vi "Is Dispense Boolean.vi"(8 "error in (no error)":errorcluster, 11 "Dispense in":refnum<class "Dispense.lvclass">) -> (0 "error out":errorcluster, 2 "Is Dispense?":bool, 3 "Dispense out":refnum<class "Dispense.lvclass">)   [LabVIEW 2016, in "Dispense.lvclass"]
uses:
  Dispense.lvclass
  Routine.lvclass
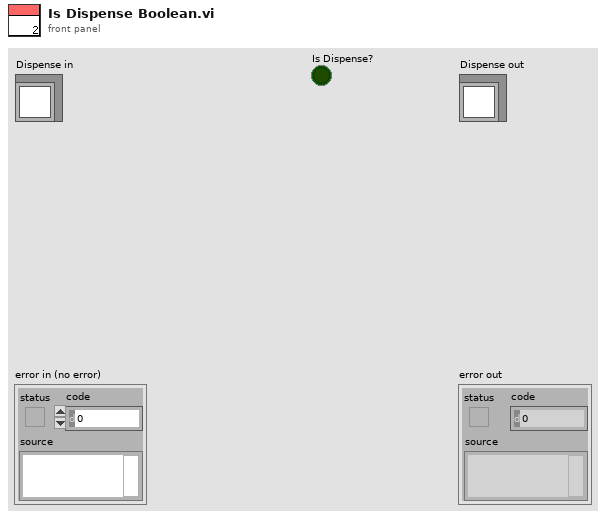
[diagram p1: front panel]
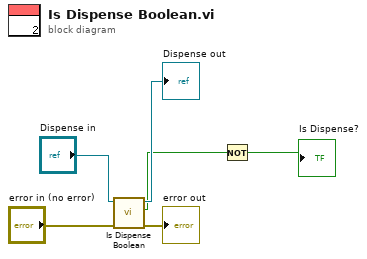
[diagram p0: block diagram]
diagram:
  n1 = call-parent "Is Dispense Boolean.vi"("error in (no error)"="error in (no error)", "Routine in"="Dispense in") -> ("error out"=→"error out":errorcluster, "Is Dispense?"=w2:bool, "Routine out"=→"Dispense out":refnum<class "Dispense.lvclass">)  [unwired: 7 in]
  n2 = Not(x=w2) -> (.not. x?=→"Is Dispense?":bool)
